vi "Build Behavior.vi"(8 "error in (no error)":errorcluster, 11 "Button Builder.lvclass":refnum<class "Button_Builder.lvclass">) -> (0 "error out":errorcluster, 2 "Panel Request Behavior":refnum<class "Panel Behavior.lvclass">, 3 "Button Builder.lvclass out":refnum<class "Button_Builder.lvclass">)   [LabVIEW 2015, in "Button_Builder.lvclass"]
uses:
  Button_Builder.lvclass
  _Depences/Panel API/Panel Request/Panle Requeset Behavior/Panel Behavior.lvclass
  Panel to Console Behaviors/Add Control in Panel/Add Control_Behavior.lvclass
  GUI Control Builder/GUI Control Builder.lvclass/GUI Control Builder.ctl
  Panel to Console Behaviors/Add Control in Panel/Add Control_Behavior.lvclass/Add Control_Behavior.ctl
  GUI Controls/GUI Control/GUI Control.lvclass
  GUI Control Builder/GUI Control Builder.lvclass
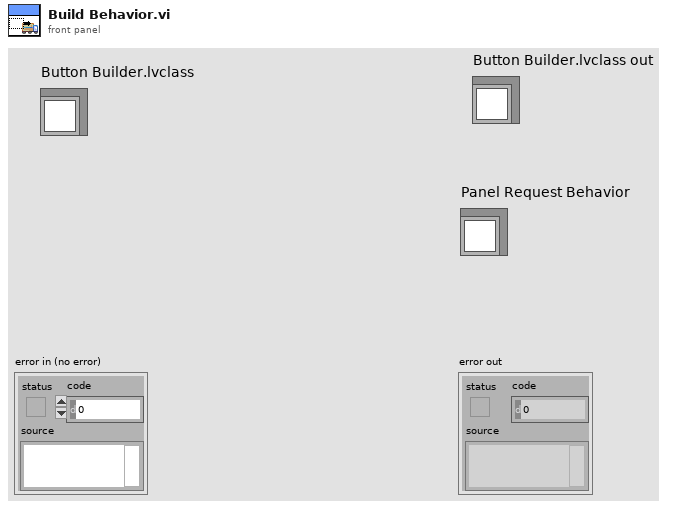
[diagram p1: front panel]
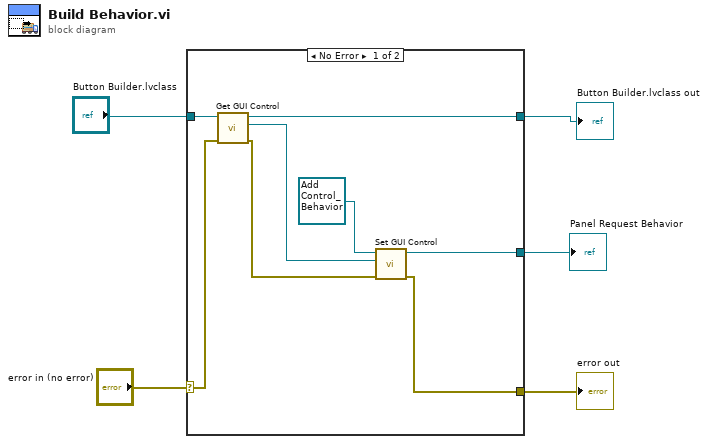
[diagram p0: block diagram]
diagram:
  n1 = case shown="No Error" "error in (no error)" {
    selector: "error in (no error)" -> [w12 w15]
    tunnel: "Button Builder.lvclass" -> [w13 w14]
    tunnel: [w9 w14] -> w1
    tunnel: [w7 _] -> w4
    tunnel: [w6 w15] -> w3
    frame No Error {
      n2 = call "Get GUI Control.vi"("error in (no error)"=w12, "Control Builder in"=w13) -> ("error out"=w10:errorcluster, "GUI Control"=w11:refnum<class "GUI Control.lvclass">, "Control Builder out"=w9:refnum<class "Button_Builder.lvclass">)  [unwired: 7 in]
      n3 = call "Set GUI Control.vi"("error in (no error)"=w10, "GUI Control"=w11, "Add Control_Behavior in"=refnum<class "Add Control_Behavior.lvclass"> refnum) -> ("error out"=w6:errorcluster, "Add Control_Behavior out"=w7:refnum<class "Add Control_Behavior.lvclass">)  [unwired: 7 in]
    }
    frame Error {
    }
  }
  "error out" <- w3
  "Panel Request Behavior" <- w4
  "Button Builder.lvclass out" <- w1
